vi "CommandDynamixelPosition.vi"(8 "error in":errorcluster, 10 "NotifierReff":T1, 11 "VISA resource name":refnum<visa-resource-name>) -> (0 "Error out":errorcluster)   [LabVIEW 2013]
uses:
  Data/TypeDefs/Notifiers.ctl
  Data/TypeDefs/UTM Location.ctl
  Data/TypeDefs/Sail Set Suggestions.ctl
  Data/TypeDefs/Rudder Set Suggestions.ctl
  Data/TypeDefs/OverrideInformation.ctl
  Data/TypeDefs/OverrideMode.ctl
  Data/TypeDefs/MotorSetup.ctl
  Data/TypeDefs/DynamixelSetupInfo.ctl
  Data/TypeDefs/AirmarStatus.ctl
  Data/TypeDefs/HardwareOnline.ctl
  Data/TypeDefs/DynamixelCycleTracker.ctl
  Data/TypeDefs/RC Input Values.ctl
  Classes/Missions/GenericMission/GenericMission.lvclass
  Classes/Waypoint/Waypoint.lvclass
panel:
  out "Written value":dbl
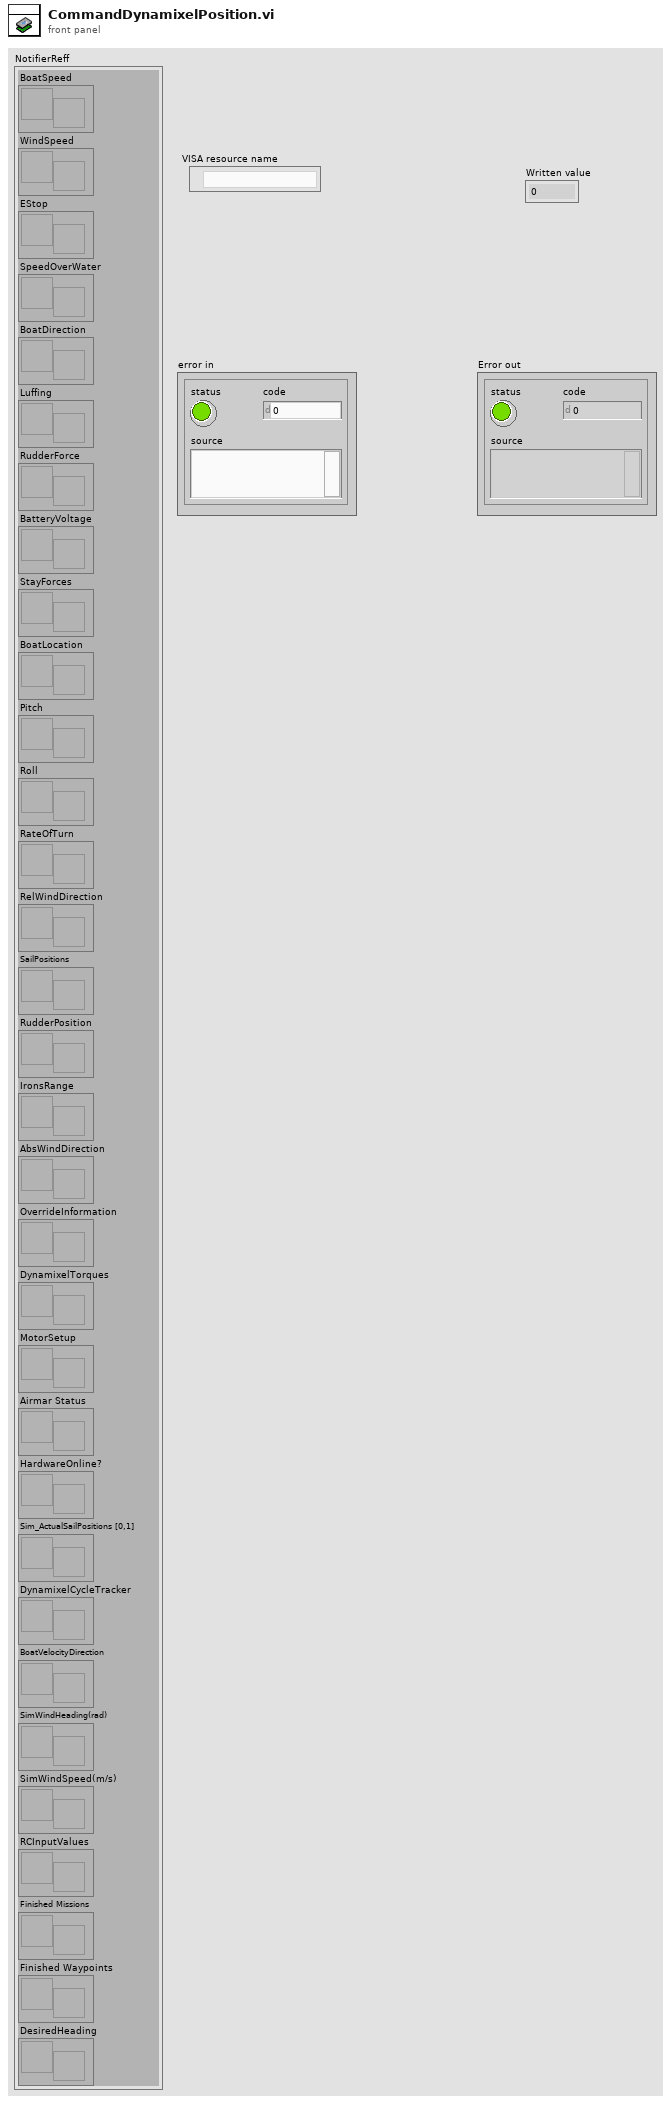
[diagram p1: front panel]
types:
  T1 = typedef "Notifiers.ctl" = cluster{"BoatSpeed":refnum<notifier>, "WindSpeed":refnum<notifier>, "EStop":refnum<notifier>, "SpeedOverWater":refnum<notifier>, "BoatDirection":refnum<notifier>, "Luffing":refnum<notifier>, "RudderForce":refnum<notifier>, "BatteryVoltage":refnum<notifier>, "StayForces":refnum<notifier>, "BoatLocation":refnum<notifier>, "Pitch":refnum<notifier>, "Roll":refnum<notifier>, "RateOfTurn":refnum<notifier>, "RelWindDirection":refnum<notifier>, "SailPositions":refnum<notifier>, "RudderPosition":refnum<notifier>, "IronsRange":refnum<notifier>, "AbsWindDirection":refnum<notifier>, "OverrideInformation":refnum<notifier>, "DynamixelTorques":refnum<notifier>, "MotorSetup":refnum<notifier>, "Airmar Status":refnum<notifier>, "HardwareOnline?":refnum<notifier>, "Sim_ActualSailPositions [0,1]":refnum<notifier>, "DynamixelCycleTracker":refnum<notifier>, "BoatVelocityDirection":refnum<notifier>, "SimWindHeading(rad)":refnum<notifier>, "SimWindSpeed(m/s)":refnum<notifier>, "RCInputValues":refnum<notifier>, "Finished Missions":refnum<notifier>, "Finished Waypoints":refnum<notifier>, "DesiredHeading":refnum<notifier>}
  T2 = typedef "Sail Set Suggestions.ctl" = cluster{"MainSailSuggestion":dbl, "JibSailSuggestion":dbl}
  T3 = typedef "Rudder Set Suggestions.ctl" = dbl
  T4 = typedef "DynamixelCycleTracker.ctl" = cluster{"Main Dynamixel\nCycle Number":i32, "Jib Dynamixel\nCycle Number":i32, "Rudder Dynamixel\nCycle Number":i32}
  T5 = typedef "MotorSetup.ctl" = cluster{"Main Dynamixel Set Data":T6, "Rudder Dynamixel Set Data":T6, "Jib Dynamixel Set Data":T6}
  T6 = typedef "DynamixelSetupInfo.ctl" = cluster{"Lower Winch Bound (deg)":dbl, "Upper Winch Bound (deg)":dbl}
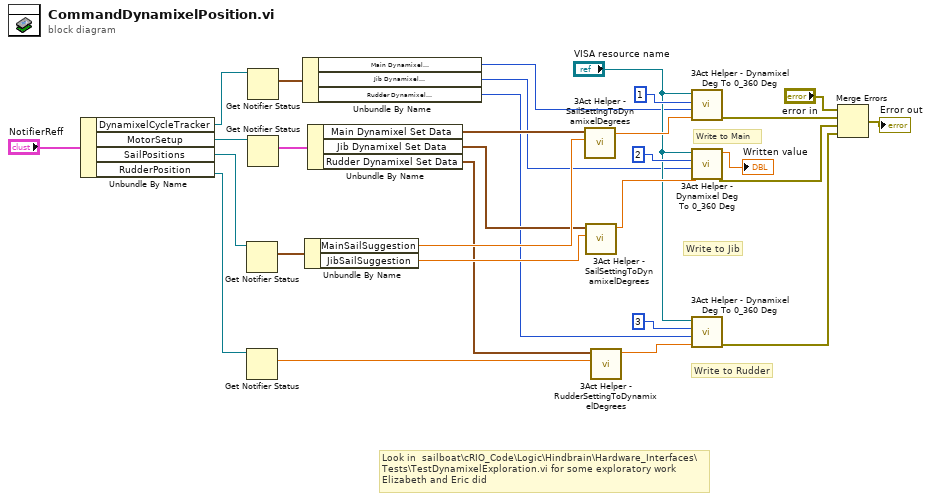
[diagram p0: block diagram]
diagram:
  # "Look in  sailboat\\cRIO_Code\\Logic\\Hindbrain\\Hardware_Interfaces\\Tests\\TestDynamixelExploration.vi for some exploratory work Elizabeth and Eric did"
  # "Write to Rudder"
  # "Write to Jib"
  # "Write to Main"
  n1 = Unbundle By Name("NotifierReff") -> ("DynamixelCycleTracker"=w6:refnum<notifier>, "MotorSetup"=w28:refnum<notifier>, "SailPositions"=w29:refnum<notifier>, "RudderPosition"=w24:refnum<notifier>)
  n2 = Get Notifier Status(notifier=w29) -> (current notification=w1:T2)  [unwired: 1 in, 4 out]
  n3 = Get Notifier Status(notifier=w24) -> (current notification=w23:T3)  [unwired: 1 in, 4 out]
  n4 = Get Notifier Status(notifier=w6) -> (current notification=w5:T4)  [unwired: 1 in, 4 out]
  n5 = Get Notifier Status(notifier=w28) -> (current notification=w27:T5)  [unwired: 1 in, 4 out]
  n6 = Unbundle By Name(w5) -> ("Main Dynamixel\nCycle Number"=w4:i32, "Jib Dynamixel\nCycle Number"=w3:i32, "Rudder Dynamixel\nCycle Number"=w2:i32)
  n7 = Unbundle By Name(w1) -> ("MainSailSuggestion"=w26:dbl, "JibSailSuggestion"=w25:dbl)
  n8 = Unbundle By Name(w27) -> ("Main Dynamixel Set Data"=w14:T6, "Jib Dynamixel Set Data"=w9:T6, "Rudder Dynamixel Set Data"=w15:T6)
  n9 = call "3Act Helper - SailSettingToDynamixelDegrees.vi"("SailSuggestion"=w26, "Dynamixel Set Data"=w14) -> ("Dynamixel Angle"=w19:dbl)  [unwired: 9 in]
  n10 = call "3Act Helper - SailSettingToDynamixelDegrees.vi"("SailSuggestion"=w25, "Dynamixel Set Data"=w9) -> ("Dynamixel Angle"=w18:dbl)  [unwired: 9 in]
  n11 = call "3Act Helper - RudderSettingToDynamixelDegrees.vi"("Suggested Rudder Setpoint"=w23, "Dynamixel Set Data"=w15) -> ("Dynamixel Angle"=w16:dbl)  [unwired: 9 in]
  n12 = call "3Act Helper - Dynamixel Deg To 0_360 Deg.vi"("Dynamixel Setpoint In (deg)"=w19, "Dynamixel Cycle Number"=w4, "Motor ID"=u8 1 ("Motor ID (0)"), "VISA resource name"="VISA resource name") -> ("Error out"=w13:errorcluster)  [unwired: 6 in, 1 out]
  n13 = call "3Act Helper - Dynamixel Deg To 0_360 Deg.vi"("Dynamixel Setpoint In (deg)"=w18, "Dynamixel Cycle Number"=w3, "Motor ID"=u8 2 ("Motor ID (0)"), "VISA resource name"="VISA resource name") -> ("Error out"=w12:errorcluster, "Written value"=→"Written value":dbl)  [unwired: 6 in]
  n14 = call "3Act Helper - Dynamixel Deg To 0_360 Deg.vi"("Dynamixel Setpoint In (deg)"=w16, "Dynamixel Cycle Number"=w2, "Motor ID"=u8 3 ("Motor ID (0)"), "VISA resource name"="VISA resource name") -> ("Error out"=w11:errorcluster)  [unwired: 6 in, 1 out]
  n15 = Merge Errors("error in", w13, w12, w11) -> (→"Error out":errorcluster)
